vi "Vehicle - Fire Station.vi"(8 "error in (no error)":errorcluster, 10 "Station":T1 max=4 step=1 scale=0.0..4.0, 11 "View Model":T2) -> (0 "error out":errorcluster, 3 "View Model":T2)   [LabVIEW 2017]
doc: "Generates user event when car move between stations"
uses:
  View Model/Controls/View Model.ctl
  View Model/Controls/Shared Model.ctl
  Error Handler/Controls/Error Model.ctl
  Error Handler/Controls/Error Data.ctl
  Error Handler/Controls/Error Level.ctl
  Configuration/Controls/Config Model.ctl
  Configuration/Controls/Config Record.ctl
  Configuration/Controls/Config Data.ctl
  Configuration/Controls/Config Command.ctl
  Controller/Controls/Controler Model.ctl
  Controls/Vehicle - Station Slider.ctl
  Controller/Controls/Controller - Wash Step.ctl
  Entry Console View/Controls/Entry Console - Wash Steps.ctl
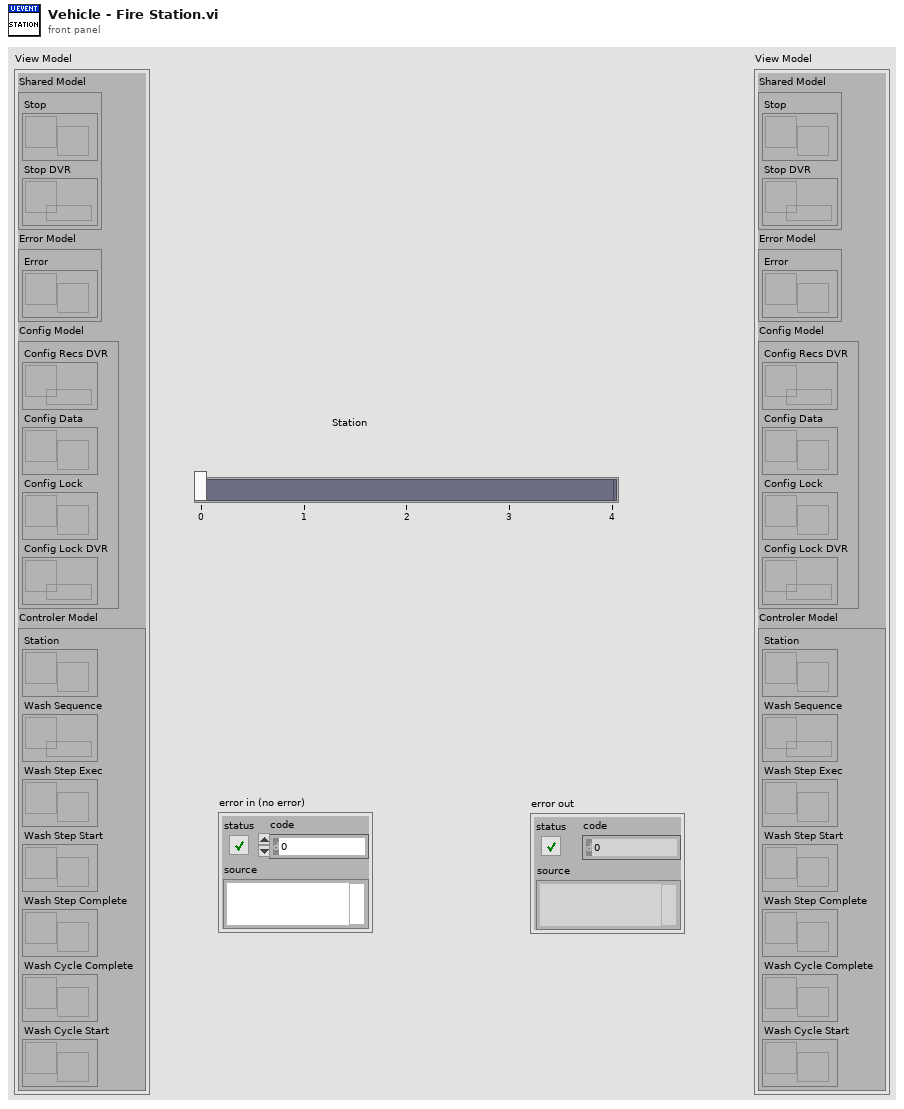
[diagram p1: front panel]
types:
  T1 = typedef "Vehicle - Station Slider.ctl" = u8
  T2 = typedef "View Model.ctl" = cluster{"Shared Model":T3, "Error Model":T4, "Config Model":T5, "Controler Model":T6}
  T3 = typedef "Shared Model.ctl" = cluster{"Stop":refnum<user-event>, "Stop DVR":refnum<data-value>}
  T4 = typedef "Error Model.ctl" = cluster{"Error":refnum<user-event>}
  T5 = typedef "Config Model.ctl" = cluster{"Config Recs DVR":refnum<data-value>, "Config Data":refnum<user-event>, "Config Lock":refnum<user-event>, "Config Lock DVR":refnum<data-value>}
  T6 = typedef "Controler Model.ctl" = cluster{"Station":refnum<user-event>, "Wash Sequence":refnum<data-value>, "Wash Step Exec":refnum<user-event>, "Wash Step Start":refnum<user-event>, "Wash Step Complete":refnum<user-event>, "Wash Cycle Complete":refnum<user-event>, "Wash Cycle Start":refnum<user-event>}
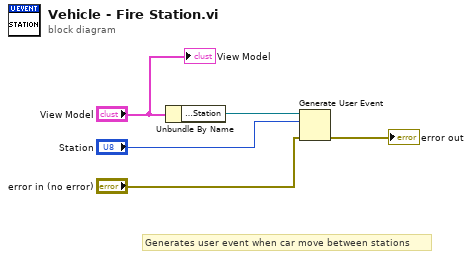
[diagram p0: block diagram]
diagram:
  # "Generates user event when car move between stations"
  n1 = Unbundle By Name("View Model") -> ("Controler Model.Station"=w5:refnum<user-event>)
  n2 = Generate User Event(user event=w5, event data cluster="Station", error in="error in (no error)") -> (error out=→"error out":errorcluster)  [unwired: 1 in, 1 out]
  "View Model" <- "View Model"
